vi "Limelight Load Pipeline.vi"(9 "Pipeline Number":dbl format="%#_13g", 11 "Load Pipeline":bool) -> ()   [LabVIEW 2020]
uses:
  <vilib>/Rock Robotics/Network Tables/NT Write Number.vi
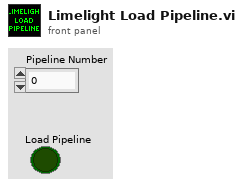
[diagram p1: front panel]
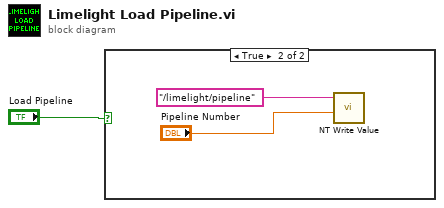
[diagram p0: block diagram]
diagram:
  n1 = case shown="True" "Load Pipeline" {
    frame False {
    }
    frame True {
      n2 = call-poly <vilib>:"NT Write Value.vi"("Numeric"="Pipeline Number", "Name"="/limelight/pipeline") -> ()  [unwired: 9 in, 1 out]
    }
  }
